vi "splitDataByChannel.vi"(8 "error in (no error)":errorcluster, 10 "Data":dbl[][](array[numeric]), 11 "K2602 in":refnum<class "K2602.lvclass">) -> (0 "error out":errorcluster, 2 "data":dbl[][][](array[numeric])=[[[0.56, 1.0], [2.0, 3.0]]], 3 "K2602 out":refnum<class "K2602.lvclass">)   [LabVIEW 2011, in "Hardware.lvlib" / "Channels.lvlib" / "K2602.lvclass"]
uses:
  K2602.lvclass
  AnalogOutput.lvclass
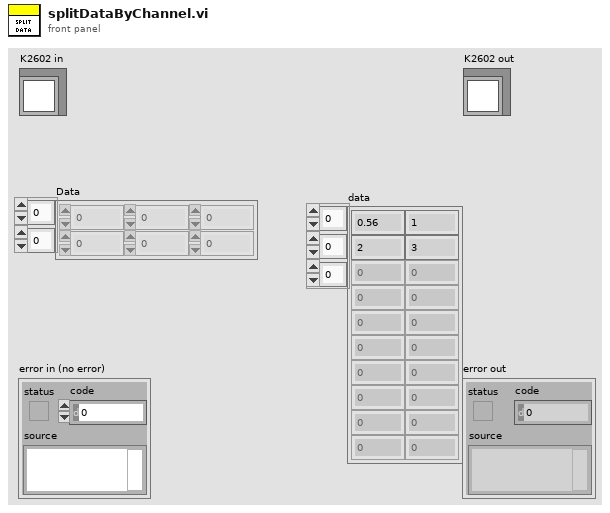
[diagram p1: front panel]
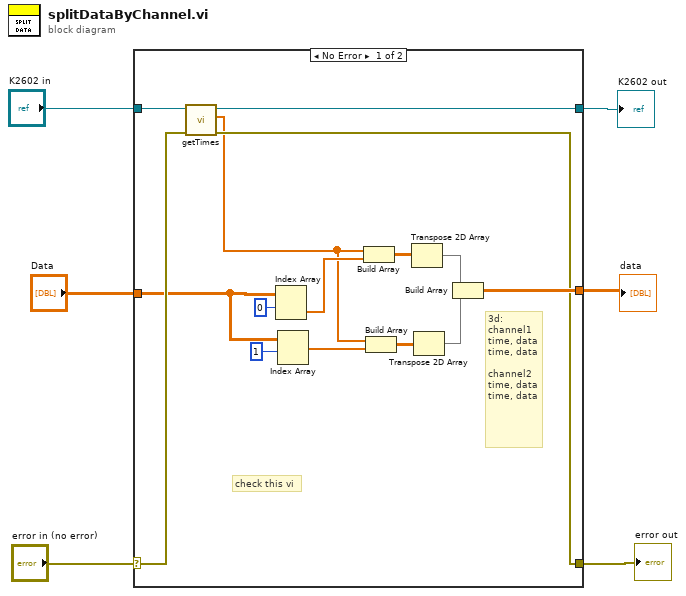
[diagram p0: block diagram]
diagram:
  n1 = case shown="No Error" "error in (no error)" {
    selector: "error in (no error)" -> [w20 w23]
    tunnel: [w12 w23] -> w5
    tunnel: [w13 w22] -> w3
    tunnel: "K2602 in" -> [w21 w22]
    tunnel: "Data" -> [w17 _]
    tunnel: [w14 _] -> w1
    frame No Error {
      # "check this vi"
      # "3d: \nchannel1\ntime, data\ntime, data\n\nchannel2\ntime, data\ntime, data"
      n2 = call "getTimes.vi"("error in (no error)"=w20, "AnalogOutput in"=w21) -> ("error out"=w12:errorcluster, "times"=w7:dbl[], "AnalogOutput out"=w13:refnum<class "K2602.lvclass">)  [unwired: 7 in]
      n3 = Index Array(array=w17, index (row)=0) -> (element=w16:dbl[])  [unwired: 1 in]
      n4 = Index Array(array=w17, index (row)=1) -> (element=w15:dbl[])  [unwired: 1 in]
      n5 = Build Array(w7, w16) -> (w11:dbl[][])
      n6 = Build Array(w7, w15) -> (w9:dbl[][])
      n7 = Transpose 2D Array(2D array=w11) -> (transposed array=w10:dbl[][])
      n8 = Transpose 2D Array(2D array=w9) -> (transposed array=w8:dbl[][])
      n9 = Build Array(w10, w8) -> (w14:dbl[][][])
    }
    frame Error {
    }
  }
  "error out" <- w5
  "K2602 out" <- w3
  "data" <- w1
